vi "SWERVE_DRIVE_GLOBALS.vi"() -> ()   [LabVIEW 2019]
uses:
  <vilib>/Rock Robotics/WPI/ThirdParty/JAS_Junk/TrajLib/TypeDef/SWERVE_DRIVE_MODULE_STATE.ctl
  <vilib>/Rock Robotics/WPI/ThirdParty/JAS_Junk/TrajLib/TypeDef/ROTATION2D.ctl
  <vilib>/Rock Robotics/WPI/ThirdParty/JAS_Junk/TrajLib/TypeDef/SWERVE_DRIVE_MODULE_POSITION.ctl
  <vilib>/Rock Robotics/WPI/ThirdParty/JAS_Junk/TrajLib/TypeDef/CHASSIS_SPEEDS.ctl
  <vilib>/Rock Robotics/WPI/ThirdParty/JAS_Junk/TrajLib/TypeDef/SWERVE_DRIVE_KINEMATICS.ctl
  <vilib>/Analysis/Matrix/Datatypes/RealMatrix.ctl
  <vilib>/Rock Robotics/WPI/ThirdParty/JAS_Junk/TrajLib/TypeDef/TRANSLATION2D.ctl
  <vilib>/Rock Robotics/WPI/ThirdParty/JAS_Junk/TrajLib/Trajectory_Library.lvlib
  <vilib>/Analysis/Matrix/NI_Matrix.lvlib
panel:
  out "Orientation_Angle_Demand_Radians":dbl format="%17.2f"
  out "Adjusted Module State Demands":T1[](array[typedef]) {"Angle"."SIN" format="%13.4f"; "Angle"."COS" format="%13.4f"; "Angle"."VALUE" format="%13.4f"}
  out "Adjusted Chassis Dmd":T3 {"vOmega" format="%10.3f"; "vY" format="%10.3f"; "vX" format="%10.3f"}
  out "SWERVE_DRIVE_KINEMATICS":T4 {"SavedModuleStates"."Angle"."SIN" format="%13.4f"; "SavedModuleStates"."Angle"."COS" format="%13.4f"; "SavedModuleStates"."Angle"."VALUE" format="%13.4f"; "PrevCoR"."Y" format="%14.3f"; "PrevCoR"."X" format="%14.3f"; "Modules"."Y" format="%14.3f"; "Modules"."X" format="%14.3f"}
  out "Swerve Chassis Speed":T3 {"vOmega" format="%10.3f"; "vY" format="%10.3f"; "vX" format="%10.3f"}
  out "Swerve Module Positions":T7[](array[typedef]) {"Angle"."SIN" format="%13.4f"; "Angle"."COS" format="%13.4f"; "Angle"."VALUE" format="%13.4f"}
  in  "Swerve Module States":T1[](array[typedef]) {"Angle"."SIN" format="%13.4f"; "Angle"."COS" format="%13.4f"; "Angle"."VALUE" format="%13.4f"}
  out "GyroHeading_Radians":dbl format="%17.2f"
  out "Mod Speed Err":dbl[](array[numeric]) format="%17.3f"
  out "Mod Wheel Out":dbl[](array[numeric]) format="%17.3f"
  out "Mod Swerve in Deadband":bool
  out "Mod Swerve On Targ":bool[](array[boolean])
  out "Mod Swerve Err":dbl[](array[numeric]) format="%17.3f"
  out "Mod Swerve Out":dbl[](array[numeric]) format="%17.3f"
  out "Orientation Correct CO":dbl format="%17.3f"
  out "Orientation Angle Error_Rad":dbl format="%17.3f"
  # "DIAGNOSTIC\nDATA"
  # "Module Drive\nSpeed"
  # "Module \nPositioning"
  # "Overall Chassis Dmd\nafter orientation correction"
  # "Orientation Correction data"
  # "Sensor Readings"
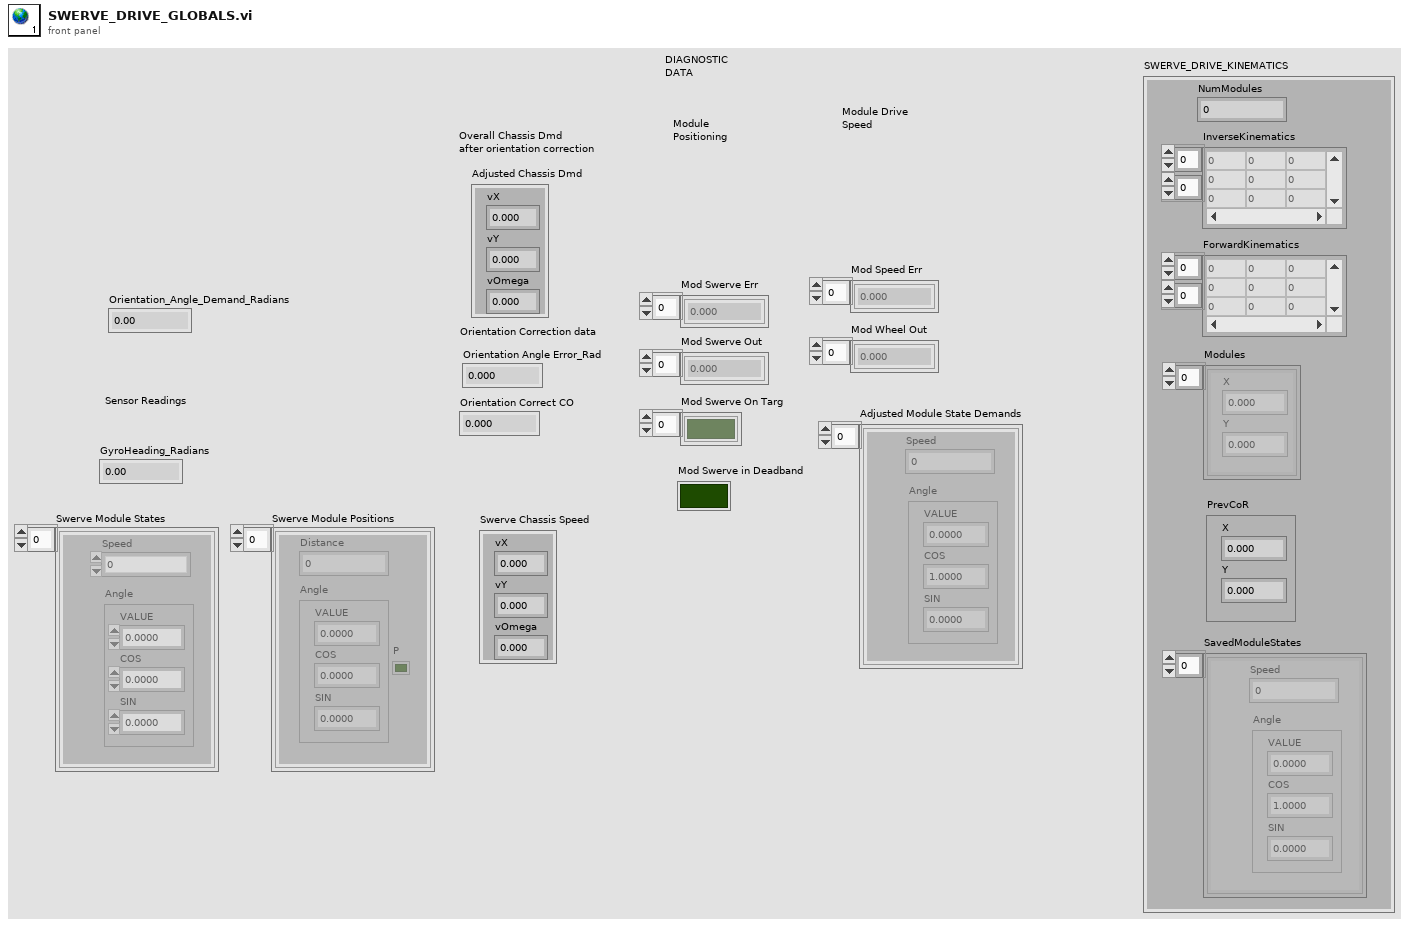
[diagram p1: front panel]
types:
  T1 = typedef "Trajectory_Library.lvlib/SWERVE_DRIVE_MODULE_STATE.ctl" = cluster{"Speed":dbl, "Angle":T2}
  T2 = typedef "Trajectory_Library.lvlib/ROTATION2D.ctl" = cluster{"VALUE":dbl, "COS":dbl, "SIN":dbl}
  T3 = typedef "Trajectory_Library.lvlib/CHASSIS_SPEEDS.ctl" = cluster{"vX":dbl, "vY":dbl, "vOmega":dbl}
  T4 = typedef "Trajectory_Library.lvlib/SWERVE_DRIVE_KINEMATICS.ctl" = cluster{"NumModules":i32, "InverseKinematics":T5, "ForwardKinematics":T5, "Modules":T6[], "PrevCoR":T6, "SavedModuleStates":T1[]}
  T5 = typedef "NI_Matrix.lvlib/RealMatrix.ctl" = dbl[][]
  T6 = typedef "Trajectory_Library.lvlib/TRANSLATION2D.ctl" = cluster{"X":dbl, "Y":dbl}
  T7 = typedef "Trajectory_Library.lvlib/SWERVE_DRIVE_MODULE_POSITION.ctl" = cluster{"Distance":dbl, "Angle":T2, "P":bool}
diagram:
